vi "CreateMutex.vi"(4 "error in (no error)":errorcluster, 5 "create if not found? (T)":bool=TRUE, 7 "name (unnamed)":string) -> (0 "error out":errorcluster, 1 "created new?":bool, 3 "hMutex":i32 format="%.0x")   [LabVIEW 2011]
uses:
  KERNEL32.DLL
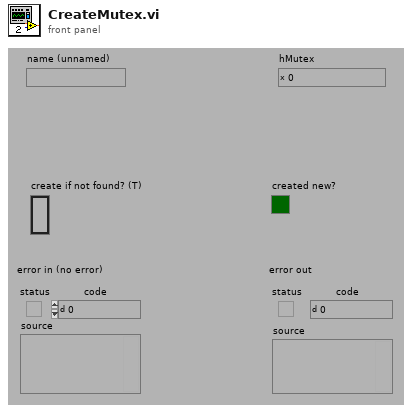
[diagram p1: front panel]
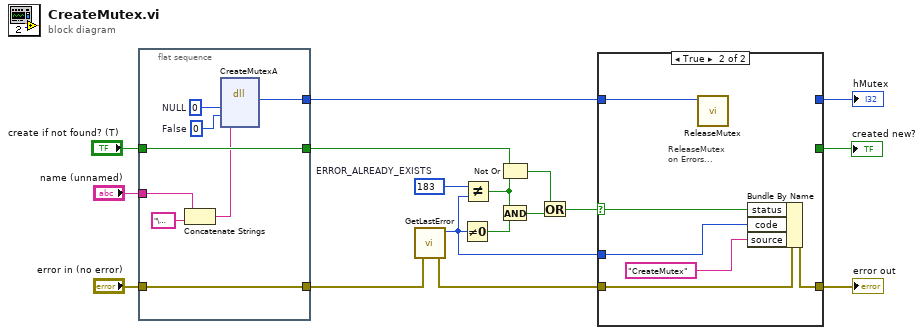
[diagram p0: block diagram]
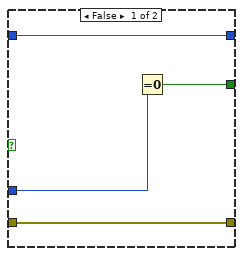
[diagram p2: hidden frame]
diagram:
  w11 = 183  # ERROR_ALREADY_EXISTS
  n1 = flat-sequence {
    tunnel: "error in (no error)" -> [w25]
    tunnel: [w25] -> w15
    tunnel: [w24] -> w12
    tunnel: "name (unnamed)" -> [w20]
    tunnel: "create if not found? (T)" -> [w22]
    tunnel: [w22] -> w1
    frame #0 {
      w21 = 0  # False
      w23 = 0  # NULL
      n2 = Concatenate Strings(w20, "\u0000" ("string")) -> (w19:string)
      n3 = dll-call lib="KERNEL32.DLL" fn="CreateMutexA" label="CreateMutex()"("lpMutexAttributes"=w23, "bInitialOwner"=w21, "lpName"=w19) -> ("hMutex"=w24:i32)  [unwired: 6 in, 2 out]
    }
  }
  n4 = call "GetLastError.vi"("error in (no error)"=w15) -> ("error out"=w17:errorcluster, "CODE"=w10:i32)  [unwired: 5 out]
  n5 = Not Equal To 0?(x=w10) -> (x != 0?=w6:bool)
  n6 = Not Equal?(x=w11, y=w10) -> (x != y?=w5:bool)
  n7 = Not Or(1:w5, 2:w1) -> (0:w8:bool)
  n8 = And(x=w5, y=w6) -> (x .and. y?=w4:bool)
  n9 = Or(x=w8, y=w4) -> (x .or. y?=w7:bool)
  n10 = case shown="True" w7 {
    selector: w7 -> [_ w34]
    tunnel: w10 -> [w27 w31]
    tunnel: w17 -> [w29 w35]
    tunnel: [w29 w33] -> w14
    tunnel: w12 -> [w28 w30]
    tunnel: [w28 _] -> w9
    tunnel: [w26 _] -> w3
    frame False {
      n11 = Equal To 0?(x=w27) -> (x = 0?=w26:bool)
    }
    frame True {
      # "ReleaseMutex\non Errors..."
      n12 = call "ReleaseMutex.vi"("hMutex (NULL)"=w30) -> ()  [unwired: 2 in, 5 out]
      n13 = Bundle By Name(cluster=w35, "status"=w34, "code"=w31, "source"="CreateMutex") -> (w33:errorcluster)
    }
  }
  "error out" <- w14
  "hMutex" <- w9
  "created new?" <- w3
